vi "Begin.vi"(8 "error in":errorcluster) -> (0 "error out":errorcluster)   [LabVIEW 2016]
doc: "Called before other user functions, this VI is expected to open initial I/O refnums, load in file data, and do all program initialization. Notice that the <B>error out</B> terminal is simply used for data flow. Wiring it to other structures or subVIs ensures that this VI runs first."
uses:
  <vilib>/Rock Robotics/WPI/DriverStation/WPI_DriverStationRobotMode2.ctl
  <vilib>/Rock Robotics/WPI/ThirdParty/CanMotor/CTRLib-LV-TalonSRX/CTRE_CANTalonSRX_ControlMode.ctl
  <vilib>/Rock Robotics/WPI/ThirdParty/CanMotor/CTRLib-LV-TalonSRX/WPI_CANTalonSRX_APIFeedbackSelect.ctl
  <vilib>/Rock Robotics/WPI/Joystick/WPI_JoystickDeviceEnum.ctl
  Robot Global Data.vi
  <vilib>/Rock Robotics/WPI/ThirdParty/Sensors/Pigeon IMU/CTRE_PigeonIMU_Open_TalonSRX.vi
  <vilib>/Rock Robotics/WPI/ThirdParty/CanMotor/CTRLib-LV-TalonSRX/Framework/CTRE_Create_SensoredGearboxDouble.vi
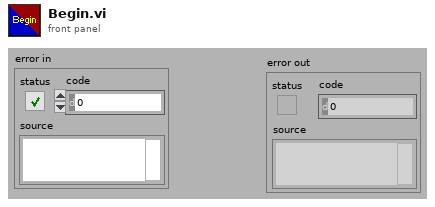
[diagram p1: front panel]
types:
  T1 = typedef "WPI_JoystickDeviceEnum.ctl" = enum16{"USB 0", "USB 1", "USB 2", "USB 3", "USB 4", "USB 5"}
  T2 = typedef "CTRE_CANTalonSRX_ControlMode.ctl" = enum16{"Throttle (Duty-Cycle)", "Position Closed-Loop", "Velocity Closed-Loop", "Current Closed-Loop", "Voltage Compensation", "Slave Follower", "Motion Profile", "Motion Magic"}
  T3 = cluster{"Wheel Radius":dbl, "Distance Between Wheels":dbl}
  T4 = typedef "WPI_CANTalonSRX_APIFeedbackSelect.ctl" = enum16{"Digital Quadrature Encoder", "Analog Potentiometer", "Analog Encoder", "Count on Quad-A (Rising-Edge)", "Count on Quad-A (Falling-Edge)", "CTR Magnetic Enc (Absolute)", "CTR Magnetic Enc (Relative)", "Pulse Width"}
  T5 = typedef "WPI_DriverStationRobotMode2.ctl" = enum16{"Autonomous Disabled", "Autonomous Enabled", "Teleop Disabled", "Teleop Enabled", "Disconnected", "Finish", "Test Disabled", "Test Enabled", "Emergency Stopped"}
  T6 = typedef "WPI_MotorControlDeviceRef.ctl" = cluster{"DeviceStatus":errorcluster, "Type":T7, "PWM":cluster{"PWM Channel":T8, "DeadBand":T9}, "CAN":cluster{"Device Number":u8, "SetOutput VI Ref":variant, "GetOutput VI Ref":variant, "Enable VI Ref":variant, "Disable VI Ref":variant, "Data":variant}, "Invert":bool}
  T7 = typedef "WPI_MotorControlType.ctl" = enum16{"PWM", "CAN"}
  T8 = typedef "FPGA_DIOPWMChannel.ctl" = enum8{"PWM 0", "PWM 1", "PWM 2", "PWM 3", "PWM 4", "PWM 5", "PWM 6", "PWM 7", "PWM 8", "PWM 9", "PWM MXP 0", "PWM MXP 1", "PWM MXP 2", "PWM MXP 3", "PWM MXP 4", "PWM MXP 5", "PWM MXP 6", "PWM MXP 7", "PWM MXP 8", "PWM MXP 9", "Invalid"}
  T9 = typedef "WPI_PWMDeadband.ctl" = cluster{"Name":string, "maxPositivePwm":i32, "minPositivePwm":i32, "centerPwm":i32, "maxNegativePwm":i32, "minNegativePwm":i32, "angularRange":u16}
  T10 = typedef "SensoredGearbox.ctl" = cluster{"Smart Motor Controller":T6, "Invert":bool, "Gear Ratio":dbl}
  T11 = typedef "WPI_JoystickDevRef.ctl" = cluster{"Device":T1}
  T12 = typedef "CTRE_PigeonIMU_DeviceRef.ctl" = cluster{"DeviceStatus":errorcluster, "Device Number":u8, "Type":T13, "Device ID":u32, "Handle":u64, "UsageFrame":u32, "Library Path":path}
  T13 = typedef "CTRE_PigeonIMU_ConnectionType.ctl" = u32
  T14 = typedef "SensoredTank.ctl" = cluster{"Sensored Gearbox Left":T10, "Sensored Gearbox Right ":T10, "Wheel Radius":dbl, "Distance Between Wheels":dbl}
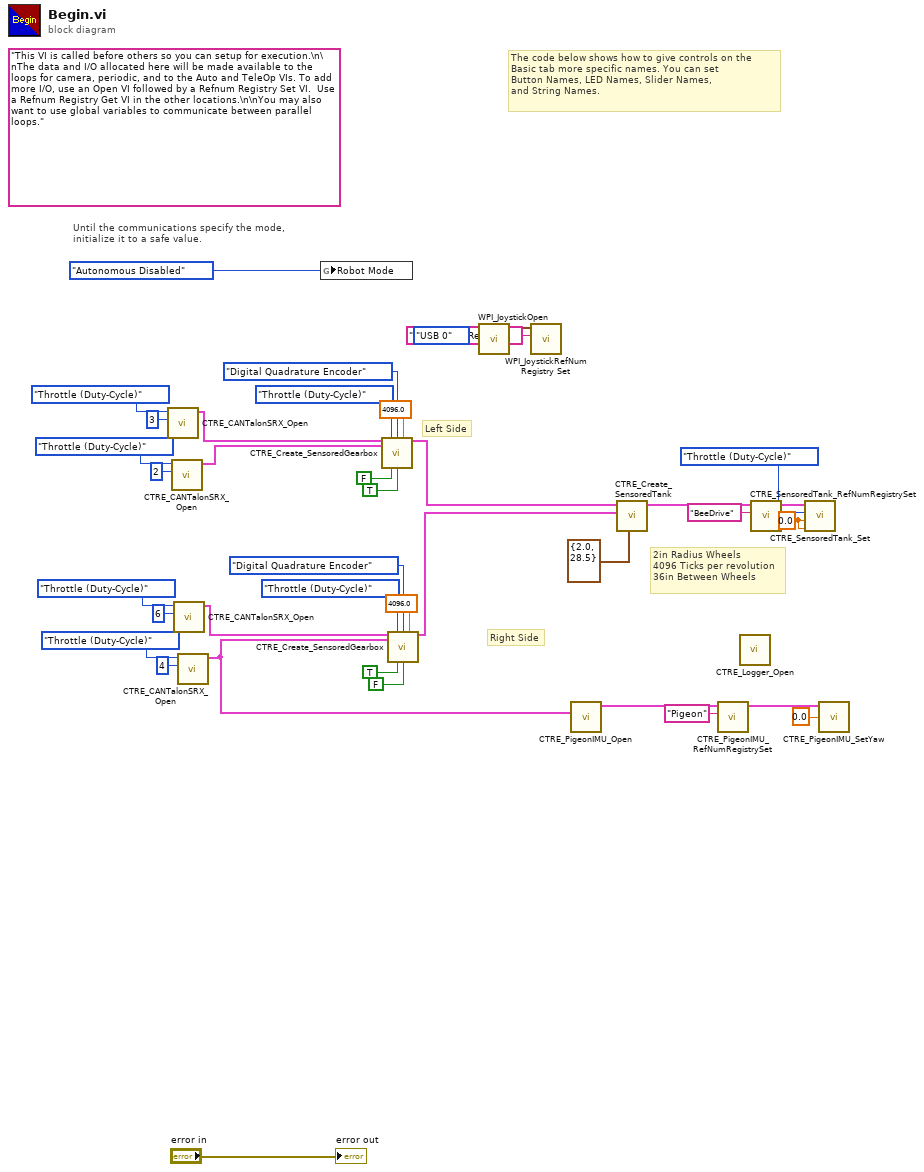
[diagram p0: block diagram]
diagram:
  w7 = 0.0 ("Forward")
  (unwired) "This VI is called before others so you can setup for execution.\n\nThe data and I/O allocated here will be made available to the loops for camera, periodic, and to the Auto and TeleOp VIs. To add more I/O, use an Open VI followed by a Refnum Registry Set VI.  Use a Refnum Registry Get VI in the other locations.\n\nYou may also want to use global variables to communicate between parallel loops."
  # "2in Radius Wheels\n4096 Ticks per revolution\n36in Between Wheels"
  # "Right Side"
  # "Left Side"
  # "The code below shows how to give controls on the\nBasic tab more specific names. You can set\nButton Names, LED Names, Slider Names,\nand String Names."
  # "Until the communications specify the mode,\ninitialize it to a safe value."
  n1 = call <vilib>:"CTRE_CANTalonSRX_Open.vi"("Device Number"=u8 3, "Control Mode"=CTRE_CANTalonSRX_ControlMode."Throttle (Duty-Cycle)") -> ("CAN Talon SRX Ref"=w33:T6)  [unwired: 8 in, 1 out]
  n2 = call <vilib>:"CTRE_CANTalonSRX_Open.vi"("Device Number"=u8 2, "Control Mode"=CTRE_CANTalonSRX_ControlMode."Throttle (Duty-Cycle)") -> ("CAN Talon SRX Ref"=w32:T6)  [unwired: 8 in, 1 out]
  n3 = call <vilib>:"CTRE_CANTalonSRX_Open.vi"("Device Number"=u8 6, "Control Mode"=CTRE_CANTalonSRX_ControlMode."Throttle (Duty-Cycle)") -> ("CAN Talon SRX Ref"=w27:T6)  [unwired: 8 in, 1 out]
  n4 = call <vilib>:"CTRE_CANTalonSRX_Open.vi"("Device Number"=u8 4, "Control Mode"=CTRE_CANTalonSRX_ControlMode."Throttle (Duty-Cycle)") -> ("CAN Talon SRX Ref"=w3:T6)  [unwired: 8 in, 1 out]
  n5 = global write "Robot Global Data.vi" "Robot Mode"(WPI_DriverStationRobotMode2."Autonomous Disabled" ("Robot Mode")) -> ()
  n6 = call-poly <vilib>:"CTRE_Create_SensoredGearbox.vi"("CAN Talon SRX Ref"=w33, "Talon SRX Control Mode"=CTRE_CANTalonSRX_ControlMode."Throttle (Duty-Cycle)", "Feedback Reference"=WPI_CANTalonSRX_APIFeedbackSelect."Digital Quadrature Encoder", "Counts Per Revolution"=4096.0 ("Gear Ratio"), "CAN Talon SRX Ref 2"=w32, "Invert"=FALSE, "Reverse Feedback Sensor"=TRUE) -> ("Sensored Gearbox"=w16:T10)  [unwired: 8 in]
  n7 = call-poly <vilib>:"CTRE_Create_SensoredGearbox.vi"("CAN Talon SRX Ref"=w27, "Talon SRX Control Mode"=CTRE_CANTalonSRX_ControlMode."Throttle (Duty-Cycle)", "Feedback Reference"=WPI_CANTalonSRX_APIFeedbackSelect."Digital Quadrature Encoder", "Counts Per Revolution"=4096.0 ("Gear Ratio"), "CAN Talon SRX Ref 2"=w3, "Invert"=TRUE, "Reverse Feedback Sensor"=FALSE) -> ("Sensored Gearbox"=w15:T10)  [unwired: 8 in]
  n8 = call <vilib>:"WPI_JoystickOpen.vi"("JoystickDevice"=WPI_JoystickDeviceEnum."USB 0") -> ("JoystickDevRef"=w5:T11)  [unwired: 10 in]
  n9 = call <vilib>:"WPI_JoystickRefNum Registry Set.vi"("refnum name"="My Joystick RefNum", "JoystickDevRef"=w5) -> ()  [unwired: 8 in, 2 out]
  n10 = call-poly <vilib>:"CTRE_PigeonIMU_Open.vi"("CAN Talon SRX Ref"=w3) -> ("PigeonIMUDevRef"=w12:T12)  [unwired: 9 in, 1 out]
  n11 = call <vilib>:"CTRE_Create_SensoredTank.vi"("Physical Features"=T3 {"Wheel Radius"=2.0, "Distance Between Wheels"=28.5}, "Sensored Gearbox Right"=w15, "Sensored Gearbox Left"=w16) -> ("Sensored Tank"=w14:T14)  [unwired: 8 in]
  n12 = call <vilib>:"CTRE_PigeonIMU_RefNumRegistrySet.vi"("refnum name"="Pigeon", "PigeonIMUDevRef"=w12) -> ("PigeonIMUDevRef"=w1:T12)  [unwired: 8 in, 1 out]
  n13 = call <vilib>:"CTRE_Logger_Open.vi"() -> ()  [unwired: 12 in]
  n14 = call <vilib>:"CTRE_SensoredTank_RefNumRegistrySet.vi"("RefNum Name"="BeeDrive", "Sensored Tank"=w14) -> ("Sensored Tank"=w9:T14)  [unwired: 9 in]
  n15 = call <vilib>:"CTRE_SensoredTank_Set.vi"("Turn"=w7, "Forward"=w7, "Talon SRX Control Mode"=CTRE_CANTalonSRX_ControlMode."Throttle (Duty-Cycle)", "Sensored Tank"=w9) -> ()  [unwired: 6 in, 2 out]
  n16 = call <vilib>:"CTRE_PigeonIMU_SetYaw.vi"("Value"=0.0, "PigeonIMUDevRef"=w1) -> ()  [unwired: 8 in, 2 out]
  "error out" <- "error in"
